vi "Setup_Dialog.vi"(11 "System Data":T4={"Core"={"Current VI Reference"=refnum, "Close Panel on Exit?"=FALSE}, "System"={"Active"=FALSE, "Exit"=FALSE, "Command wait"="", "Status_Time"=0}, "Stepper Motor"={"Connection Reference"="", "Valid Connection"=FALSE, "Speed"=15}, "Camera Data"={"Image path"=path "", "Filenames"=[], "Filenames queue"=[]}} {"Stepper Motor"."Speed" scale=0.0..30.0}) -> (3 "System Data out":T1={"Core"={"Current VI Reference"=refnum, "Close Panel on Exit?"=FALSE}, "System"={"Active"=FALSE, "Exit"=FALSE, "Command wait"="", "Status_Time"=0}, "Stepper Motor"={"Sensitivity"=0.031415926535897934, "Connection Reference"="", "Valid Connection"=FALSE}, "Camera Data"={"Image path"=path "", "Filenames"=[], "Filenames queue"=[]}} {"Stepper Motor"."Sensitivity" min=0.0 step=0.031415926535897934})   [LabVIEW 2019]
uses:
  System Data.ctl
  Stepper Data.ctl
  Camera Data.ctl
panel:
  in  "Image folder":path caption="Path"
  in  "Cancel":bool
  in  "OK":bool
  in  "Focus Sensitivity":dbl[unit]=0.15707963267948966 caption="Numeric" min=0.0 step=0.031415926535897934
  # "/step"
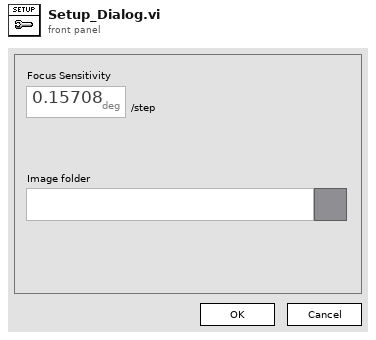
[diagram p1: front panel]
types:
  T1 = typedef "System Data.ctl" = cluster{"Core":cluster{"Current VI Reference":refnum<vi>, "Close Panel on Exit?":bool}, "System":cluster{"Active":bool, "Exit":bool, "Command wait":string, "Status_Time":i32}, "Stepper Motor":T2, "Camera Data":T3}
  T2 = typedef "Stepper Data.ctl" = cluster{"Sensitivity":dbl[unit], "Connection Reference":refnum<visa-resource-name>, "Valid Connection":bool}
  T3 = typedef "Camera Data.ctl" = cluster{"Image path":path, "Filenames":string[], "Filenames queue":string[]}
  T4 = typedef "System Data.ctl" = cluster{"Core":cluster{"Current VI Reference":refnum<vi>, "Close Panel on Exit?":bool}, "System":cluster{"Active":bool, "Exit":bool, "Command wait":string, "Status_Time":i32}, "Stepper Motor":T5, "Camera Data":T3}
  T5 = typedef "Stepper Data.ctl" = cluster{"Connection Reference":refnum<visa-resource-name>, "Valid Connection":bool, "Speed":i32}
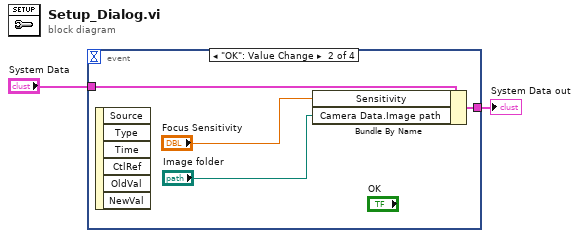
[diagram p0: block diagram]
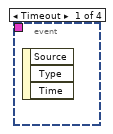
[diagram p2: hidden frame]
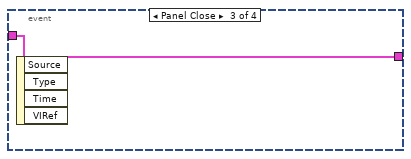
[diagram p3: hidden frame]
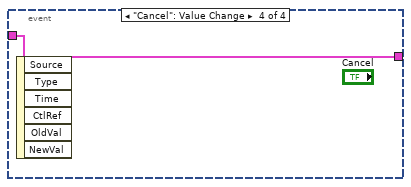
[diagram p4: hidden frame]
diagram:
  n1 = event shown="[1] \"OK\": Value Change" {
    selector: _ -> [_ _ _ _]
    dyn-events: _ -> [_ _ _ _]
    timeout: _ -> [_ _ _ _]
    tunnel: [_ w6 w7 w8] -> w1
    tunnel: "System Data" -> [_ w4 w7 w8]
    event Timeout {
      n2 = event-data() -> ()  [unwired: 1 in, 3 out]
    }
    event "OK": Value Change {
      n3 = event-data() -> ()  [unwired: 1 in, 6 out]
      n4 = Bundle By Name(cluster=w4, "Sensitivity"="Focus Sensitivity", "Camera Data.Image path"="Image folder") -> (w6:T4)
    }
    event Panel Close {
      n5 = event-data() -> ()  [unwired: 1 in, 4 out]
    }
    event "Cancel": Value Change {
      n6 = event-data() -> ()  [unwired: 1 in, 6 out]
    }
  }
  "System Data out" <- w1
